vi "Error Log AE.vi"(7 "Command":T1, 8 "error in (no error)":errorcluster, 11 "error Message":errorcluster) -> (0 "error out":errorcluster)   [LabVIEW 2016, in "Error Log.lvlib"]
uses:
  Error Log.lvlib
  Error Log Command.ctl
  User Interface/Create Path Command.ctl
  <vilib>/Utility/file.llb/Write Delimited Spreadsheet (string).vi
  User Interface/User Interface.lvlib
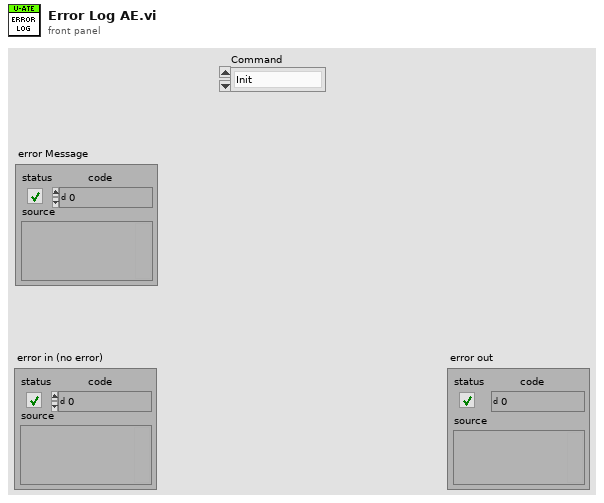
[diagram p1: front panel]
types:
  T1 = typedef "Error Log.lvlib/Error Log Command.ctl" = enum16{"Init", "Read", "Write", "Close"}
  T2 = typedef "User Interface.lvlib/Create Path Command.ctl" = enum16{"Authentication", "Hardware", "Configuration", "Calibration", "Instrument", "Test Description", "Data", "Report", "Action log", "Error Log"}
  T3 = enum16{"open", "replace", "create", "open or create", "replace or create", "replace or create with confirmation"}
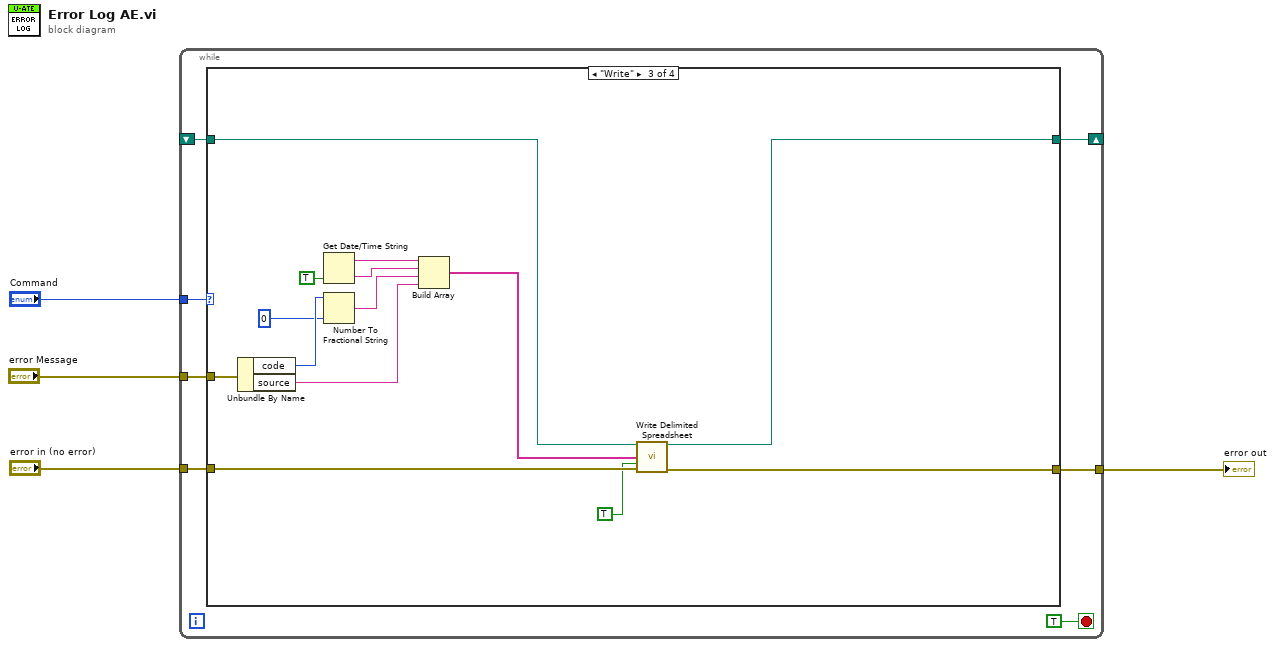
[diagram p0: block diagram]
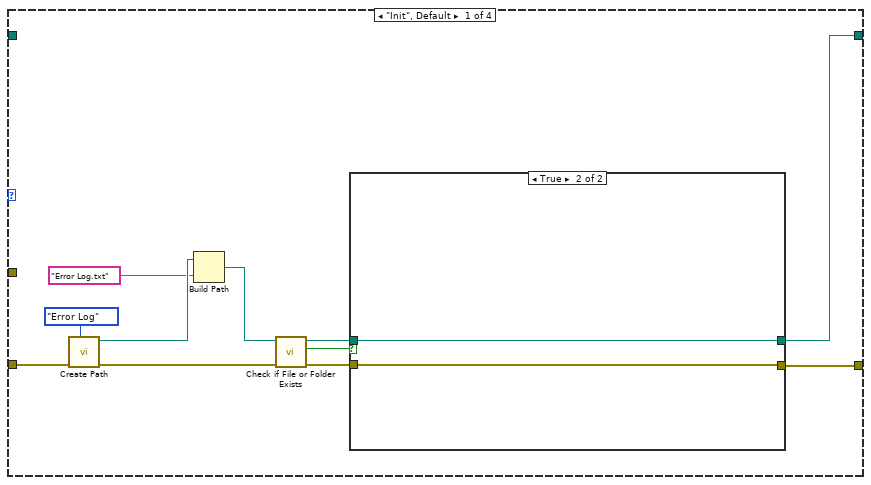
[diagram p2: hidden frame]
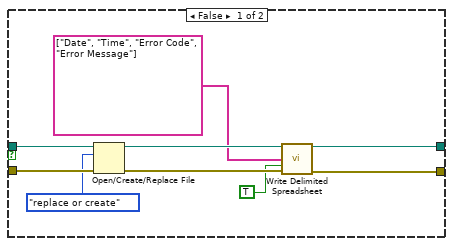
[diagram p3: hidden frame]
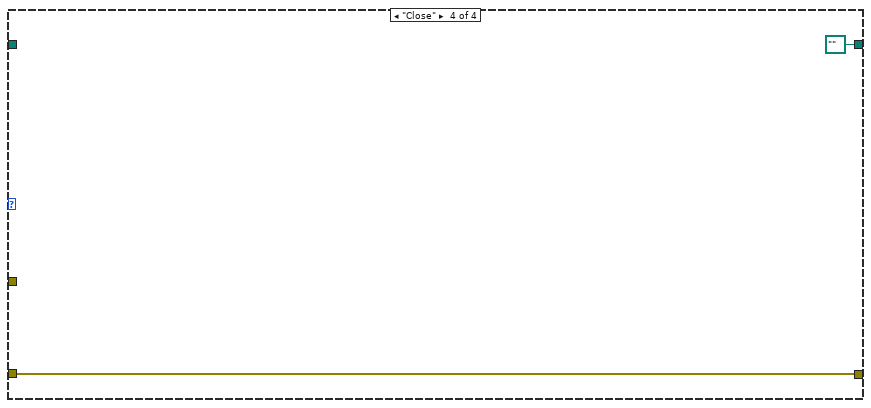
[diagram p5: hidden frame]
diagram:
  n1 = while {
    tunnel: "error in (no error)" -> [w10]
    tunnel: "Command" -> [w9]
    tunnel: [w8] -> w2
    shift-right: [w7] -> _
    shift-left: _ -> [w6]
    tunnel: "error Message" -> [w5]
    stop <- TRUE stop-if-true
    n2 = case shown="\"Write\"" w9 {
      tunnel: w10 -> [w22 w33 w47 w49]
      tunnel: [w13 w33 w46 w49] -> w8
      tunnel: [w12 w34 w43 path "" ("new file path (Not A Path if cancelled)")] -> w7
      tunnel: w6 -> [_ w34 w44 _]
      tunnel: w5 -> [_ _ w42 _]
      frame "Init", Default {
        n3 = call "Create Path.vi"("Path Command"=Create_Path_Command."Error Log", "error in (no error)"=w22) -> ("error out"=w18:errorcluster, "created path"=w20:path)  [unwired: 8 in]
        n4 = Build Path(base path=w20, name or relative path="Error Log.txt") -> (appended path=w17:path)
        n5 = call <vilib>:"Check if File or Folder Exists.vi"("error in (no error)"=w18, "path"=w17) -> ("error out"=w16:errorcluster, "file or folder exists?"=w15:bool, "dup path"=w14:path)  [unwired: 7 in]
        n6 = case shown="True" w15 {
          tunnel: w16 -> [w30 w31]
          tunnel: w14 -> [w28 w32]
          tunnel: [w26 w32] -> w12
          tunnel: [w25 w31] -> w13
          frame False {
            n7 = Open/Create/Replace File(file path (use dialog)=w28, error in=w30, operation (0:open)=T3."replace or create") -> (error out=w27:errorcluster)  [unwired: 3 in, 2 out]
            n8 = call-poly <vilib>:"Write Delimited Spreadsheet.vi"("file path (dialog if empty)"=w28, "1D data"=string[] ["Date", "Time", "Error Code", "Error Message"], "append to file? (new file:F)"=TRUE, "error in (no error)"=w27) -> ("new file path (Not A Path if cancelled)"=w26:path, "error out"=w25:errorcluster)  [unwired: 10 in]
          }
          frame True {
          }
        }
      }
      frame "Read" {
      }
      frame "Write" {
        n9 = Unbundle By Name(w42) -> ("code"=w41:i32, "source"=w36:string)
        n10 = Get Date/Time String(want seconds? (F)=TRUE) -> (date string=w39:string, time string=w38:string)  [unwired: 2 in]
        n11 = Number To Fractional String(number=w41, precision (6)=i16 0) -> (F-format string=w37:string)  [unwired: 2 in]
        n12 = Build Array(w39, w38, w37, w36) -> (w35:string[])
        n13 = call-poly <vilib>:"Write Delimited Spreadsheet.vi"("file path (dialog if empty)"=w44, "1D data"=w35, "append to file? (new file:F)"=TRUE, "error in (no error)"=w47) -> ("new file path (Not A Path if cancelled)"=w43:path, "error out"=w46:errorcluster)  [unwired: 10 in]
      }
      frame "Close" {
      }
    }
  }
  "error out" <- w2
